vi "SUB_COM_INIT.vi"(2 "baud rate (9600)":u32=9600, 3 "VISA resource name":refnum<visa-resource-name>) -> (0 "error out":errorcluster, 1 "VISA resource name out":refnum<visa-resource-name>)   [LabVIEW 2011]
uses:
  <vilib>/Instr/_visa.llb/VISA Configure Serial Port (Instr).vi
panel:
  out "Numeric":i32
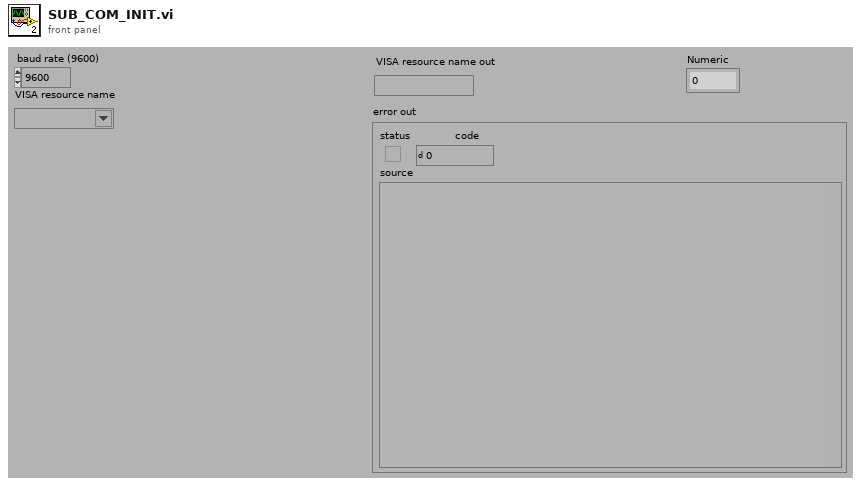
[diagram p1: front panel]
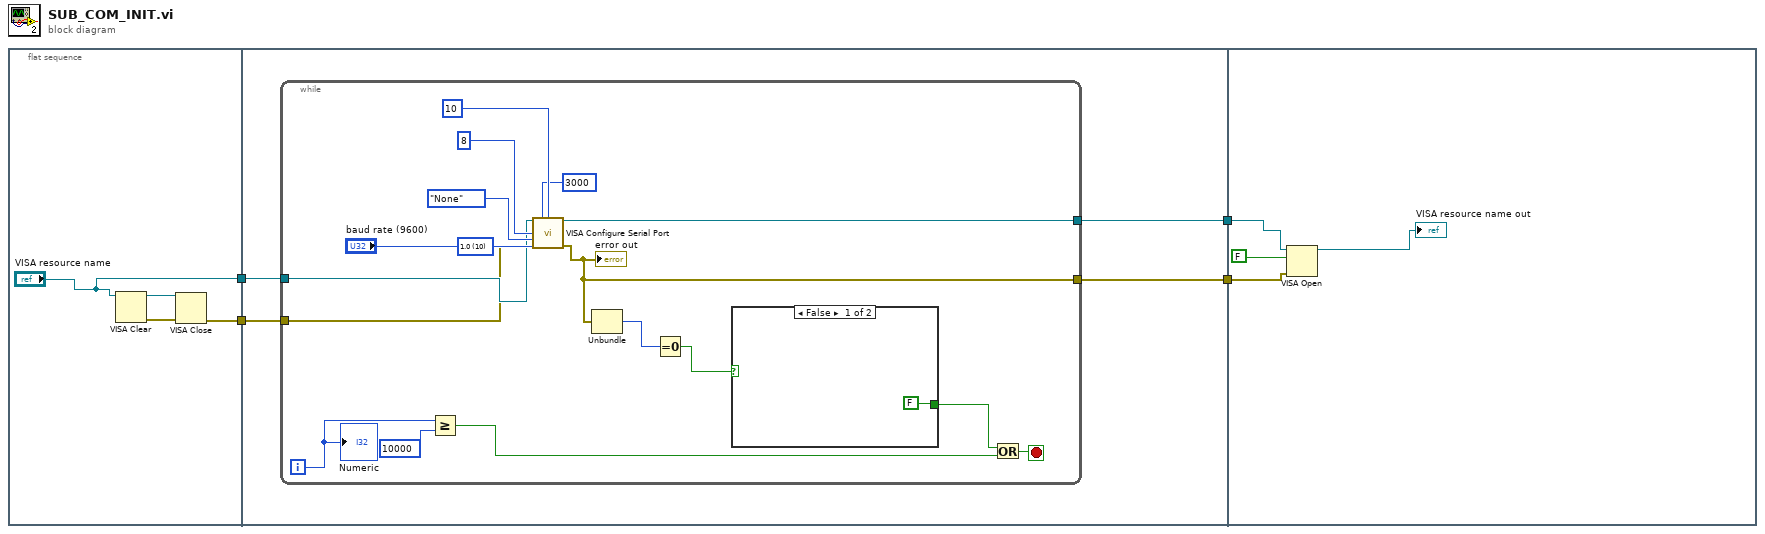
[diagram p0: block diagram]
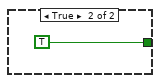
[diagram p2: hidden frame]
diagram:
  n1 = flat-sequence {
    tunnel: ["VISA resource name"] -> w2
    tunnel: [w5] -> w1
    tunnel: [w12] -> w4
    tunnel: [w11] -> w3
    tunnel: w2 -> [w10]
    tunnel: w1 -> [w9]
    tunnel: w4 -> [w33]
    tunnel: w3 -> [w32]
    frame #0 {
      n2 = VISA Clear(VISA resource name="VISA resource name") -> (VISA resource name out=w7:refnum<visa-resource-name>, error out=w8:errorcluster)  [unwired: 1 in]
      n3 = VISA Close(VISA resource name=w7, error in (no error)=w8) -> (error out=w5:errorcluster)
    }
    frame #1 {
      n4 = while {
        tunnel: [w21] -> w12
        tunnel: [w18] -> w11
        tunnel: w10 -> [w14]
        tunnel: w9 -> [w13]
        i -> [w17]
        stop <- w20 stop-if-true
        w27 = u16 10 items=["1.0"=10, "1.5"=15, "2.0"=20] ("stop bits (10: 1 bit)")
        n5 = Greater Or Equal?(x=w17, y=10000) -> (x >= y?=w16:bool)
        n6 = call-poly "VISA Configure Serial Port"("VISA resource name"=w14, "timeout (10sec)"=u32 3000, "termination char\n(0xA = '\\n' = LF)"=u8 10 ("termination char\n(0xA = '\\n' = LF)"), "baud rate (9600)"="baud rate (9600)", "data bits (8)"=u16 8, "parity (0:none)"=enum16{"None", "Odd", "Even", "Mark", "Space"}."None", "error in (no error)"=w13, "stop bits (10: 1 bit)"=w27) -> ("VISA resource name out"=w21:refnum<visa-resource-name>, "error out"=w18:errorcluster)  [unwired: 6 in]
        "error out" <- w18
        n7 = Unbundle(w18) -> ("code"=w23:i32)  [unwired: 2 out]
        n8 = Equal To 0?(x=w23) -> (x = 0?=w22:bool)
        n9 = case shown="False" w22 {
          tunnel: [FALSE TRUE] -> w19
          frame False {
          }
          frame True {
          }
        }
        n10 = Or(x=w19, y=w16) -> (x .or. y?=w20:bool)
        "Numeric" <- w17
      }
    }
    frame #2 {
      n11 = VISA Open(duplicate session (F)=FALSE, error in (no error)=w32, VISA resource name=w33) -> (VISA resource name=→"VISA resource name out":refnum<visa-resource-name>)  [unwired: 2 in, 1 out]
    }
  }
